vi "Enclose in Structure - Parse Structure Type.vi"(8 "error in":errorcluster, 11 "QD Text":string) -> (0 "error out":errorcluster, 3 "Structure Type":T1=enum."For Loop")   [LabVIEW 2020]
uses:
  Enclose in Structure - Structure Type.ctl
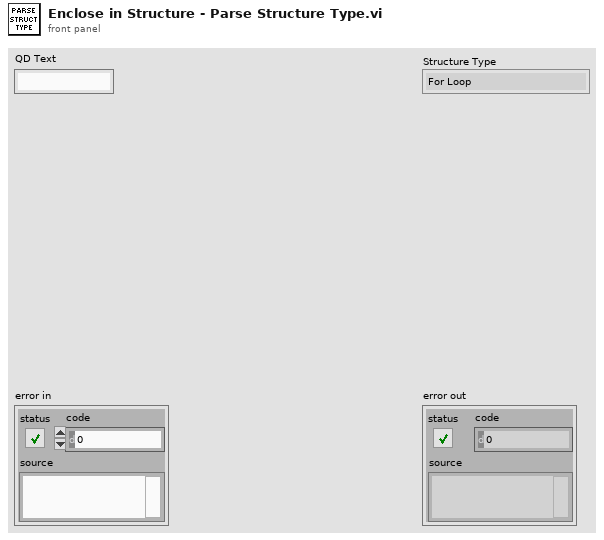
[diagram p1: front panel]
types:
  T1 = typedef "Enclose in Structure - Structure Type.ctl" = enum16{"<Invalid>", "For Loop", "While Loop", "Timed Loop", "Timed Sequence", "Case Structure", "Event Structure", "In Place Element Structure", "Flat Sequence", "Diagram Disable Structure", "Conditional Disable Structure", "Type Specialization Structure"}
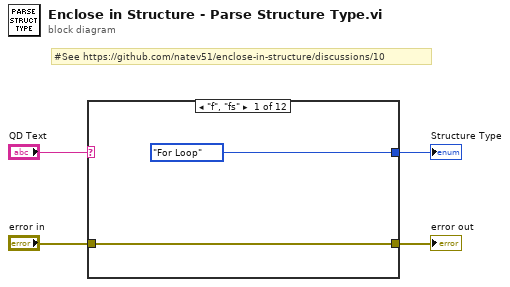
[diagram p0: block diagram]
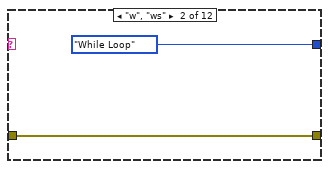
[diagram p2: hidden frame]
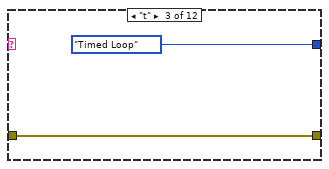
[diagram p3: hidden frame]
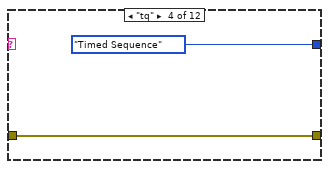
[diagram p4: hidden frame]
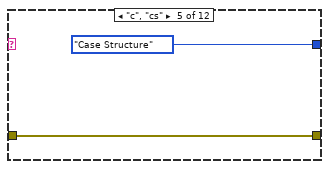
[diagram p5: hidden frame]
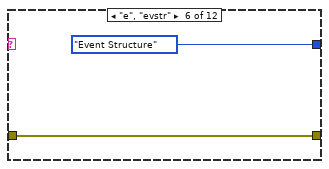
[diagram p6: hidden frame]
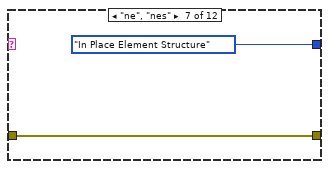
[diagram p7: hidden frame]
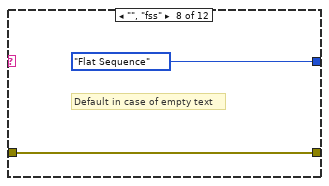
[diagram p8: hidden frame]
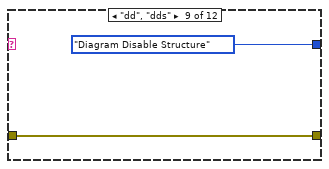
[diagram p9: hidden frame]
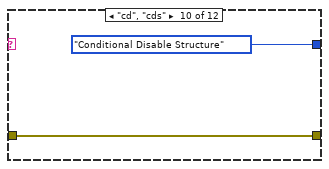
[diagram p10: hidden frame]
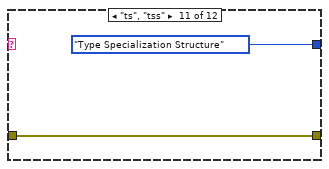
[diagram p11: hidden frame]
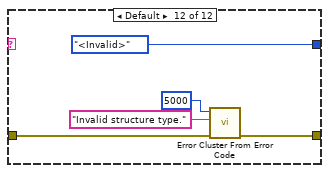
[diagram p12: hidden frame]
diagram:
  # "#See https://github.com/natev51/enclose-in-structure/discussions/10"
  n1 = case shown="\"f\", \"fs\"" "QD Text" {
    tunnel: "error in" -> [w5 w7 w9 w11 w13 w15 w17 w19 w21 w23 w25 w28]
    tunnel: [w5 w7 w9 w11 w13 w15 w17 w19 w21 w23 w25 w29] -> w3
    tunnel: [Enclose_in_Structure_-_Structure_Type."For Loop" ("Structure Type") Enclose_in_Structure_-_Structure_Type."While Loop" ("Structure Type") Enclose_in_Structure_-_Structure_Type."Timed Loop" ("Structure Type") Enclose_in_Structure_-_Structure_Type."Timed Sequence" ("Structure Type") Enclose_in_Structure_-_Structure_Type."Case Structure" ("Structure Type") Enclose_in_Structure_-_Structure_Type."Event Structure" ("Structure Type") Enclose_in_Structure_-_Structure_Type."In Place Element Structure" ("Structure Type") Enclose_in_Structure_-_Structure_Type."Flat Sequence" ("Structure Type") Enclose_in_Structure_-_Structure_Type."Diagram Disable Structure" ("Structure Type") Enclose_in_Structure_-_Structure_Type."Conditional Disable Structure" ("Structure Type") Enclose_in_Structure_-_Structure_Type."Type Specialization Structure" ("Structure Type") Enclose_in_Structure_-_Structure_Type."<Invalid>" ("Structure Type")] -> w2
    frame "f", "fs" {
    }
    frame "w", "ws" {
    }
    frame "t" {
    }
    frame "tq" {
    }
    frame "c", "cs" {
    }
    frame "e", "evstr" {
    }
    frame "ne", "nes" {
    }
    frame "", "fss" {
      # "Default in case of empty text"
    }
    frame "dd", "dds" {
    }
    frame "cd", "cds" {
    }
    frame "ts", "tss" {
    }
    frame Default {
      n2 = call <vilib>:"Error Cluster From Error Code.vi"("error in (no error)"=w28, "error message (\"\")"="Invalid structure type." ("error message (\"\")"), "error code (0)"=5000) -> ("error out"=w29:errorcluster)  [unwired: 6 in]
    }
  }
  "error out" <- w3
  "Structure Type" <- w2
